vi "PayloadData_ToCluster.vi"(8 "error in":errorcluster, 10 "Payload Read":string="20.60,10.00,22,OFF,173.08,0") -> (0 "error out":errorcluster, 2 "Sensor Data Cluster Out":T1)   [LabVIEW 2024]
uses:
  Controls/SensorDataCluster.ctl
panel:
  in  "use system decimal point (T)":bool=TRUE
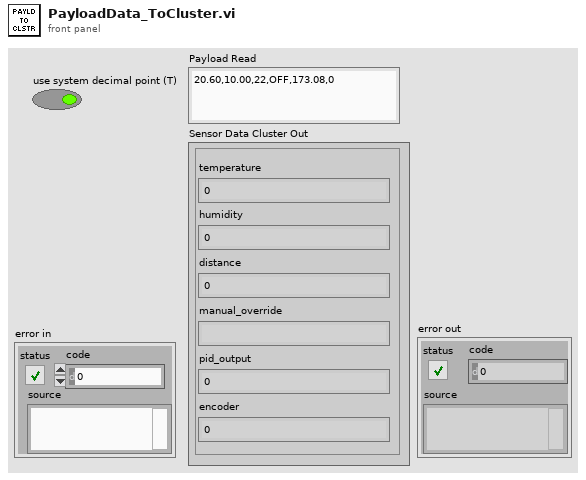
[diagram p1: front panel]
types:
  T1 = typedef "SensorDataCluster.ctl" = cluster{"temperature":dbl, "humidity":dbl, "distance":dbl, "manual_override":string, "pid_output":dbl, "encoder":dbl}
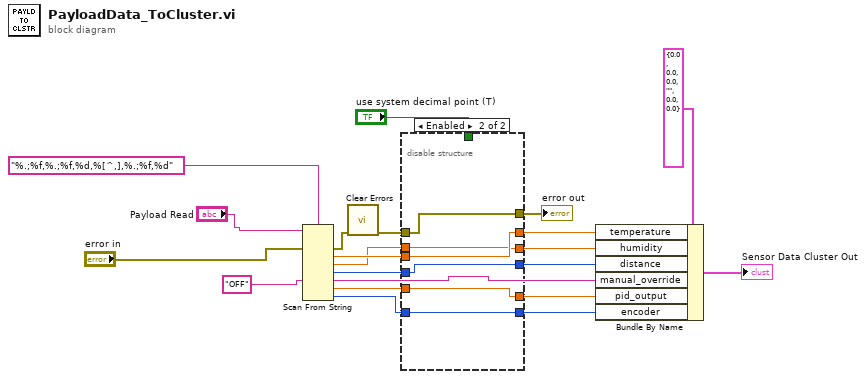
[diagram p0: block diagram]
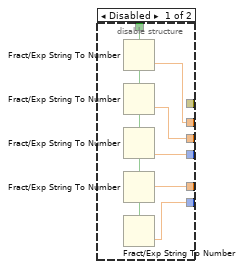
[diagram p2: hidden frame]
diagram:
  n1 = Scan From String(format string="%.;%f,%.;%f,%d,%[^,],%.;%f,%d", input string="Payload Read", error in="error in", default 4="OFF" ("default value 4")) -> (error out=w3:errorcluster, output 1=w10:dbl, output 2=w9:dbl, output 3=w8:i32, output 4=w11:string, output 5=w7:dbl, output 6=w6:i32)  [unwired: 6 in, 2 out]
  n2 = call <vilib>:"Clear Errors.vi"("error in (no error)"=w3) -> ("error out"=w1:errorcluster)  [unwired: 5 in, 1 out]
  n3 = disable-structure shown="Enabled" {
    disable-tunnel: [w27 w29] -> w17
    disable-tunnel: [w26 w30] -> w16
    disable-tunnel: [w25 w31] -> w15
    disable-tunnel: [w24 w32] -> w14
    disable-tunnel: [w23 w33] -> w13
    disable-tunnel: "use system decimal point (T)" -> [w22 _]
    disable-tunnel: w10 -> [_ w33]
    disable-tunnel: w9 -> [_ w32]
    disable-tunnel: w8 -> [_ w31]
    disable-tunnel: w7 -> [_ w30]
    disable-tunnel: w6 -> [_ w29]
    disable-tunnel: [_ w28] -> w2
    disable-tunnel: w1 -> [_ w28]
    frame Disabled {
      n4 = Fract/Exp String To Number(use system decimal point (T)=w22) -> (number=w23:dbl)  [unwired: 3 in, 1 out]
      n5 = Fract/Exp String To Number(use system decimal point (T)=w22) -> (number=w24:dbl)  [unwired: 3 in, 1 out]
      n6 = Fract/Exp String To Number(use system decimal point (T)=w22) -> (number=w25:dbl)  [unwired: 3 in, 1 out]
      n7 = Fract/Exp String To Number(use system decimal point (T)=w22) -> (number=w26:dbl)  [unwired: 3 in, 1 out]
      n8 = Fract/Exp String To Number(use system decimal point (T)=w22) -> (number=w27:dbl)  [unwired: 3 in, 1 out]
    }
    frame Enabled {
    }
  }
  "error out" <- w2
  n9 = Bundle By Name(cluster=T1 {"temperature"=0.0, "humidity"=0.0, "distance"=0.0, "manual_override"="", "pid_output"=0.0, "encoder"=0.0} ("Sensor Data Cluster"), "temperature"=w13, "humidity"=w14, "distance"=w15, "manual_override"=w11, "pid_output"=w16, "encoder"=w17) -> (→"Sensor Data Cluster Out":T1)
